vi "Label Message.vi"(8 "error in (no error)":errorcluster, 10 "Label":string, 11 "Message":refnum<class "MSG.lvclass">) -> (0 "error out":errorcluster, 3 "Message":refnum<class "MSG.lvclass">)   [LabVIEW 2011, in "Messenging.lvlib" / "MSG.lvclass"]
uses:
  MSG.lvclass
  MSG.lvclass/MSG.ctl
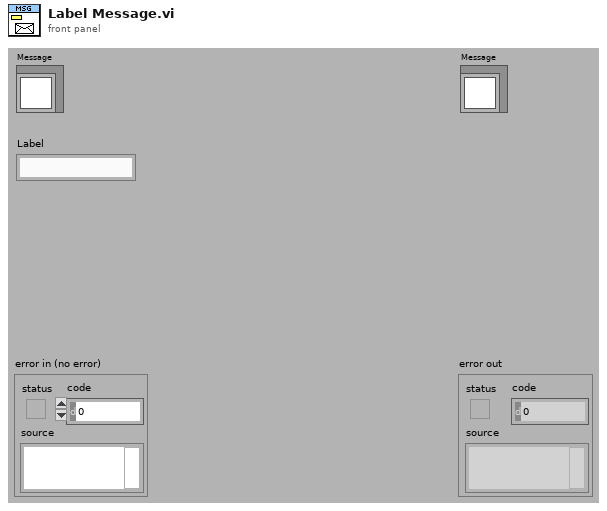
[diagram p1: front panel]
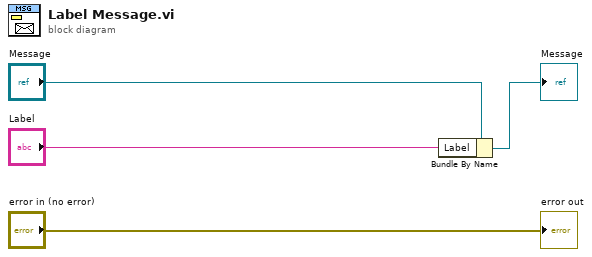
[diagram p0: block diagram]
diagram:
  n1 = Bundle By Name(cluster="Message", "Label"="Label") -> (→"Message":refnum<class "MSG.lvclass">)
  "error out" <- "error in (no error)"
